vi "Do.vi"(8 "error in":errorcluster, 10 "Actor in":refnum<class "Actor.lvclass">, 11 "Update CVT Data":refnum<class "Update CVT Data.lvclass">) -> (0 "error out":errorcluster, 2 "Actor out":refnum<class "Actor.lvclass">)   [LabVIEW 2014, in "Controller.lvlib" / "Update CVT Data.lvclass"]
doc: "(<B>Filename</B>: Actor Framework.lvlib:Message.lvclass:Do.vi)\n\nDefines what a message does when it is received by an actor. Generally, a message instructs an actor to invoke one of its methods. By default, this method does nothing. A child class must override it to define behavior. Create a child class by using the Actor Framework Message Maker dialog box."
uses:
  Update CVT Data.lvclass
  <vilib>/ActorFramework/Actor/Actor.lvclass
  Update CVT Data.lvclass/Update CVT Data.ctl
  Controller.lvclass
  SuperActor/Ex Nested.lvclass/Ex Nested.ctl
  SuperActor/Read CVT Session.vi
  SuperActor/Read Log Session.vi
  <userlib>/_Session Fwk/Session - Root.lvclass
  reusable/Session APIs/CVT/CVT.lvclass
  reusable/Session APIs/Session Log/System Log.lvclass
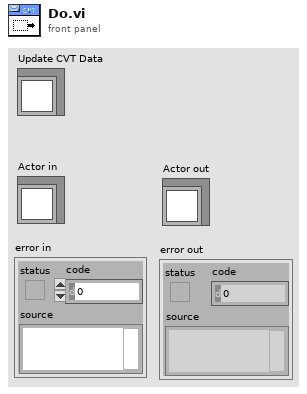
[diagram p1: front panel]
types:
  T1 = typedef "Session - Root.lvclass/Session Handle.ctl" = refnum<data-value>
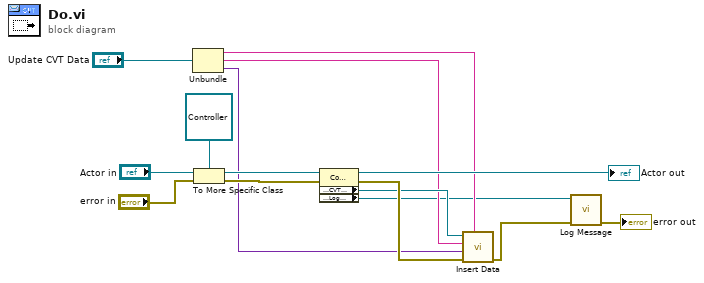
[diagram p0: block diagram]
diagram:
  n1 = Unbundle("Update CVT Data") -> (w7:string, w4:string, w5:variant)
  n2 = To More Specific Class(target class=refnum<class "Controller.lvclass"> refnum ("Controller.lvlib:Controller"), reference="Actor in", error in="error in") -> (specific class reference=w11:refnum<class "Controller.lvclass">, error out=w9:errorcluster)
  n3 = property class="Controller"(reference=w11, error in=w9) -> (reference out=→"Actor out":refnum<class "Controller.lvclass">, error out=w8:errorcluster, "Accessors:CVT Session"=w6:T1, "Accessors:Log Session"=w3:T1)
  n4 = call "Insert Data.vi"("Group"=w7, "error in"=w8, "Data"=w5, "tag"=w4, "CVT Session In"=w6) -> ("error out"=w2:errorcluster)  [unwired: 5 in, 1 out]
  n5 = call "Log Message.vi"("error in"=w2, "session in"=w3) -> ("error out"=→"error out":errorcluster)  [unwired: 8 in, 1 out]
